vi "Database.Main.vi"() -> ()   [LabVIEW 2016]
uses:
  Database.Main.Action.ctl
  Database.Main.Data.ctl
  Database.Main.Data.Status.ctl
  Database.Main.Data.Sets.ctl
  Database.Main.Data.Results.ctl
  ProdaNG/Controls/ProdaNG.Identification.ctl
  ProdaNG/Controls/ProdaNG.ProcessResult.ctl
  ProdaNG/Controls/ProdaNG.ProcessStepResult.ctl
  ProdaNG/Controls/ProdaNG.TestStepResult.ctl
  ProdaNG/Controls/ProdaNG.TestValueResult.ctl
  Database.Main.Data.Variant.ctl
  ProdaNG/Controls/ProdaNG.ProcessStepParam.ctl
  ProdaNG/Controls/ProdaNG.TestStep.ctl
  ProdaNG/Controls/ProdaNG.TestStepParam.ctl
  ProdaNG/Controls/ProdaNG.TestValue.ctl
  tools/CitTemplate/citTemplate.errData.ctl
  tools/EventLog/EventLog.EventSource.ctl
  Databaser.SelectVariant.Format.ctl
  Logger/Logger.FileBody.ctl
  CheckStatusData.ctl
  Database.Global.vi
panel:
  out "Data out":T1 {"Variant"."TS"."TV"."minimum" format="%#.3f"; "Variant"."TS"."TV"."maximum" format="%#.3f"; "Variant"."TS"."TP"."value" format="%#.3f"}
  out "error.action":string
  out "error":errorcluster
  out "_loop":i32(ring)=4
  out "action":T15=enum."--- DB ---"
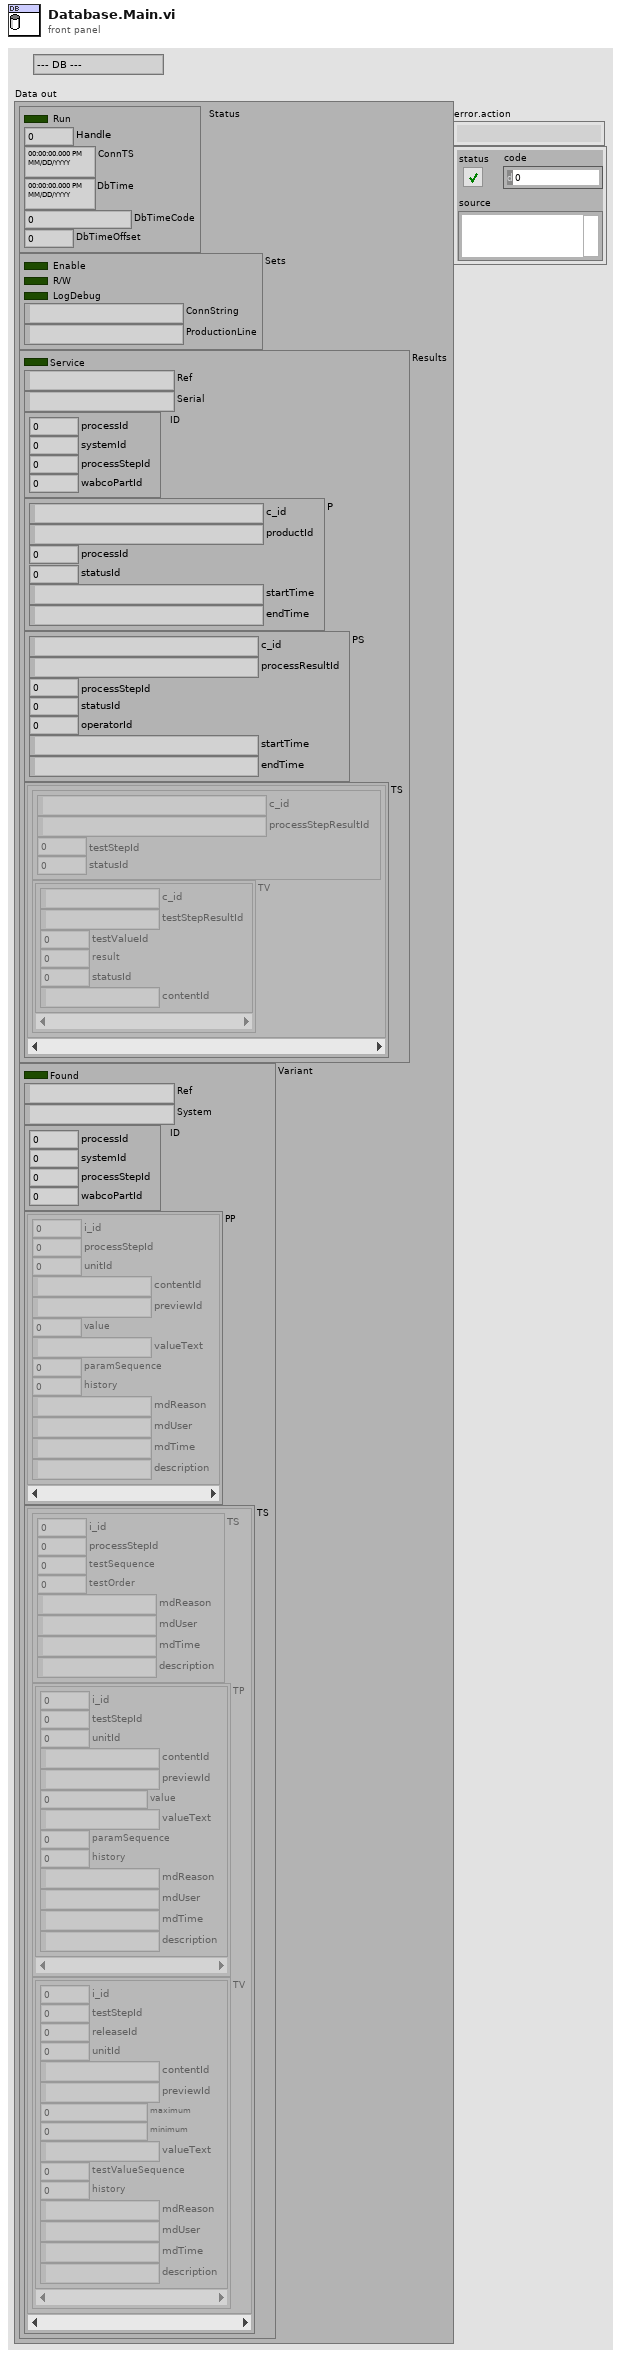
[diagram p1: front panel]
types:
  T1 = typedef "Database.Main.Data.ctl" = cluster{"Status":T2, "Sets":T3, "Results":T4, "Variant":T10}
  T2 = typedef "Database.Main.Data.Status.ctl" = cluster{"Run":bool, "Handle":i32, "ConnTS":timestamp, "DbTime":timestamp, "DbTimeCode":dbl, "DbTimeOffset":dbl}
  T3 = typedef "Database.Main.Data.Sets.ctl" = cluster{"Enable":bool, "R/W":bool, "LogDebug":bool, "ConnString":string, "ProductionLine":string}
  T4 = typedef "Database.Main.Data.Results.ctl" = cluster{"Service":bool, "Ref":string, "Serial":string, "ID":T5, "P":T6, "PS":T7, "TS":cluster{"TS":T8, "TV":T9[]}[]}
  T5 = typedef "ProdaNG.Identification.ctl" = cluster{"processId":i32, "systemId":i32, "processStepId":i32, "wabcoPartId":i32}
  T6 = typedef "ProdaNG.ProcessResult.ctl" = cluster{"c_id":string, "productId":string, "processId":i32, "statusId":i32, "startTime":string, "endTime":string}
  T7 = typedef "ProdaNG.ProcessStepResult.ctl" = cluster{"c_id":string, "processResultId":string, "processStepId":i32, "statusId":i32, "operatorId":i32, "startTime":string, "endTime":string}
  T8 = typedef "ProdaNG.TestStepResult.ctl" = cluster{"c_id":string, "processStepResultId":string, "testStepId":i32, "statusId":i32}
  T9 = typedef "ProdaNG.TestValueResult.ctl" = cluster{"c_id":string, "testStepResultId":string, "testValueId":i32, "result":dbl, "statusId":i32, "contentId":string}
  T10 = typedef "Database.Main.Data.Variant.ctl" = cluster{"Found":bool, "Ref":string, "System":string, "ID":T5, "PP":T11[], "TS":cluster{"TS":T12, "TP":T13[], "TV":T14[]}[]}
  T11 = typedef "ProdaNG.ProcessStepParam.ctl" = cluster{"i_id":i32, "processStepId":i32, "unitId":i32, "contentId":string, "previewId":string, "value":dbl, "valueText":string, "paramSequence":i32, "history":i32, "mdReason":string, "mdUser":string, "mdTime":string, "description":string}
  T12 = typedef "ProdaNG.TestStep.ctl" = cluster{"i_id":i32, "processStepId":i32, "testSequence":i32, "testOrder":i32, "mdReason":string, "mdUser":string, "mdTime":string, "description":string}
  T13 = typedef "ProdaNG.TestStepParam.ctl" = cluster{"i_id":i32, "testStepId":i32, "unitId":i32, "contentId":string, "previewId":string, "value":dbl, "valueText":string, "paramSequence":i32, "history":i32, "mdReason":string, "mdUser":string, "mdTime":string, "description":string}
  T14 = typedef "ProdaNG.TestValue.ctl" = cluster{"i_id":i32, "testStepId":i32, "releaseId":i32, "unitId":i32, "contentId":string, "previewId":string, "maximum":dbl, "minimum":dbl, "valueText":string, "testValueSequence":i32, "history":i32, "mdReason":string, "mdUser":string, "mdTime":string, "description":string}
  T15 = typedef "Database.Main.Action.ctl" = enum32{"idle", "constructor", "destructor", "--- DB ---", "Init", "Setup", "Select.Variant", "File.Export", "UpdateVariantFiles", "CheckStatus"}
  T16 = typedef "citTemplate.errData.ctl" = cluster{"ts":timestamp, "src":T17, "instance":i32, "action":string, "error":errorcluster, "unconfirmed":bool}
  T17 = typedef "EventLog.EventSource.ctl" = enum16{"All", "Gui", "Ref", "File", "Arch", "Seq", "CPX", "DB", "Laser", "Scan.P", "Scan.O", "PLC"}
  T18 = typedef "Databaser.SelectVariant.Format.ctl" = cluster{"System":string, "Variant":string}
  T19 = typedef "Logger.FileBody.ctl" = cluster{"Path":path, "System":string, "Status":u8, "Ref1":string, "Serial1":string, "Ref2":string, "Serial2":string, "Values":sgl[]}
  T20 = typedef "CheckStatusData.ctl" = cluster{"system":string, "Variant":string, "Serial":string}
  T21 = typedef "citTemplate.notifierHandle.ctl" = refnum<notifier>
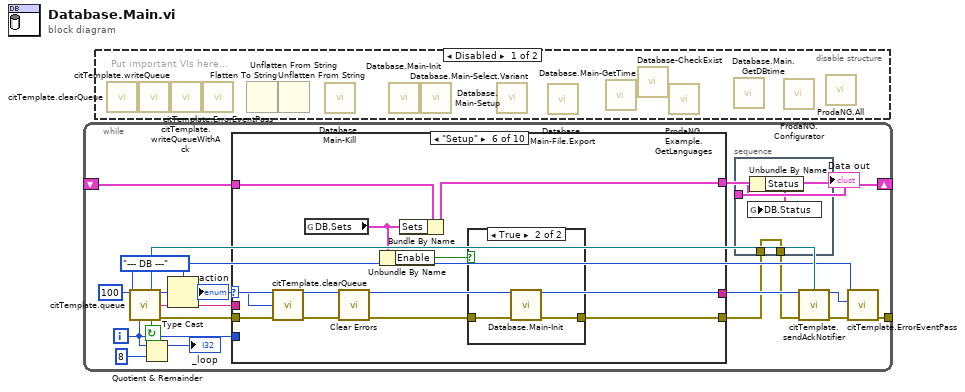
[diagram p0: block diagram]
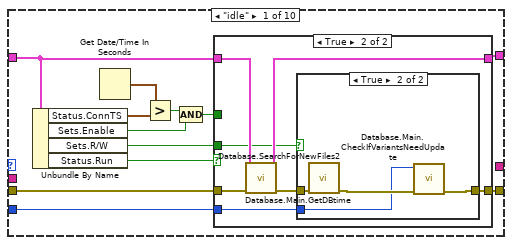
[diagram p3: hidden frame]
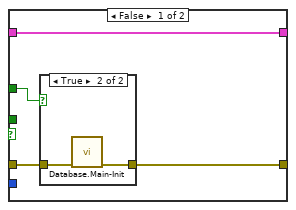
[diagram p4: hidden frame]
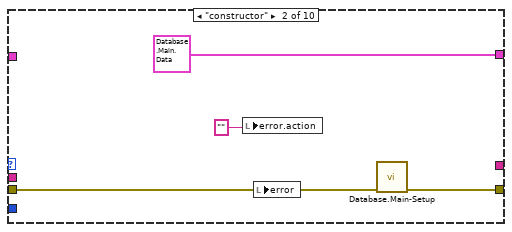
[diagram p7: hidden frame]
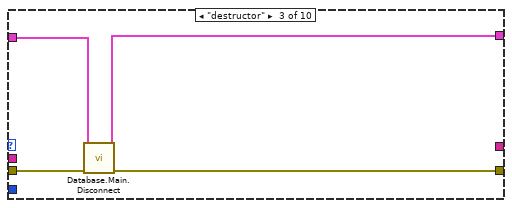
[diagram p8: hidden frame]
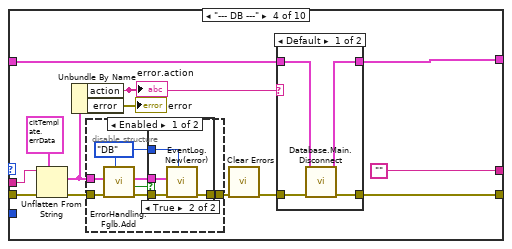
[diagram p9: hidden frame]
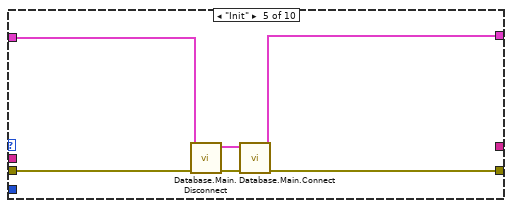
[diagram p13: hidden frame]
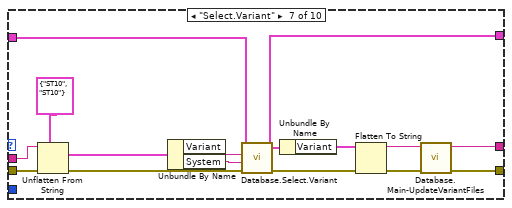
[diagram p15: hidden frame]
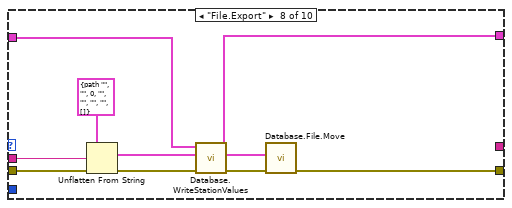
[diagram p16: hidden frame]
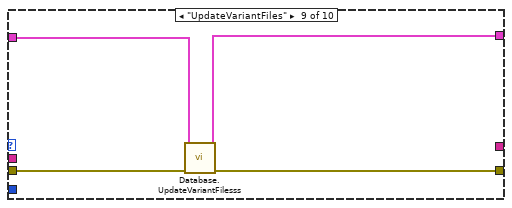
[diagram p17: hidden frame]
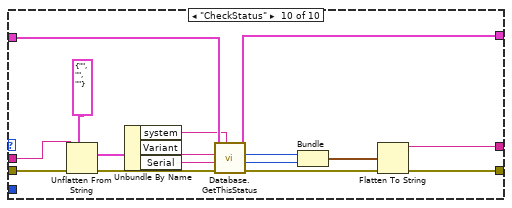
[diagram p18: hidden frame]
diagram:
  n1 = while {
    tunnel: [w12] -> _
    shift-right: [w2] -> _
    shift-left: _ -> [w3]
    i -> [w1]
    stop <- w14 continue-if-true
    w6 = Database.Main.Action."--- DB ---" ("Action")
    n2 = call "citTemplate.queue.vi"("ms timeout (250 ms)"=100, "event enum"=w6, "iteration (-1)"=w1) -> ("notifierHandle out"=w7:T21, "event out"=w17:u32, "(flatten) data out"=w16:string, "continue"=w14:bool, "error out"=w15:errorcluster)  [unwired: 2 in, 6 out]
    n3 = Quotient & Remainder(x=w1, y=8) -> (x-y*floor(x/y)=→"_loop":i32)  [unwired: 1 out]
    n4 = Type Cast(type=w6, x=w17) -> (*(type *) &x=w11:T15)
    "action" <- w11
    n5 = case shown="\"Setup\"" w11 {
      selector: w11 -> [_ _ _ _ _ w104 _ _ _ _]
      tunnel: w16 -> [_ _ _ w67 _ _ w121 w128 _ w136]
      tunnel: w15 -> [w30 w53 w59 w72 w94 w105 w122 w127 w135 w142]
      tunnel: [w27 w55 w58 w69 w96 w101 w113 w130 w134 w146] -> w5
      tunnel: w3 -> [w26 _ w57 w70 w93 w100 w119 w131 w133 w151]
      tunnel: [_ _ _ "" _ _ w117 _ _ w144] -> w8
      tunnel: [w22 T1 {"Status"={"Run"=FALSE, "Handle"=0, "ConnTS"=timestamp(0 s since 1904-01-01), "DbTime"=timestamp(0 s since 1904-01-01), "DbTimeCode"=0.0, "DbTimeOffset"=0.0}, "Sets"={"Enable"=FALSE, "R/W"=FALSE, "LogDebug"=FALSE, "ConnString"="", "ProductionLine"=""}, "Results"={"Service"=FALSE, "Ref"="", "Serial"="", "ID"={"processId"=0, "systemId"=0, "processStepId"=0, "wabcoPartId"=0}, "P"={"c_id"="", "productId"="", "processId"=0, "statusId"=0, "startTime"="", "endTime"=""}, "PS"={"c_id"="", "processResultId"="", "processStepId"=0, "statusId"=0, "operatorId"=0, "startTime"="", "endTime"=""}, "TS"=[]}, "Variant"={"Found"=FALSE, "Ref"="", "System"="", "ID"={"processId"=0, "systemId"=0, "processStepId"=0, "wabcoPartId"=0}, "PP"=[], "TS"=[]}} ("Data") w56 w60 w91 w97 w115 w123 w132 w150] -> w2
      tunnel: w1 -> [w21 _ _ _ _ _ _ _ _ _]
      frame "idle" {
        n6 = Unbundle By Name(w26) -> ("Status.ConnTS"=w31:timestamp, "Sets.Enable"=w24:bool, "Sets.R/W"=w23:bool, "Status.Run"=w28:bool)
        n7 = Get Date/Time In Seconds() -> (seconds since 1Jan1904=w32:timestamp)
        n8 = Greater?(x=w32, y=w31) -> (0:w29:bool)
        n9 = Compound Arithmetic op=AND(w29, w24) -> (w25:bool)
        n10 = case shown="True" w28 {
          tunnel: w30 -> [w36 w44]
          tunnel: w25 -> [w35 _]
          tunnel: [w34 w42] -> w27
          tunnel: w26 -> [w33 w46]
          tunnel: [w33 w45] -> w22
          tunnel: w23 -> [_ w41]
          tunnel: w21 -> [_ w40]
          frame False {
            n11 = case shown="True" w35 {
              tunnel: w36 -> [w37 w39]
              tunnel: [w37 w38] -> w34
              frame False {
              }
              frame True {
                n12 = call "Database.Main-Init.vi"("error in"=w39) -> ("error out"=w38:errorcluster)  [unwired: 10 in]
              }
            }
          }
          frame True {
            n13 = call "Database.Main.GetDBtime.vi"("error in (no error)"=w44, "Data in"=w46) -> ("error out"=w43:errorcluster, "Data out"=w45:T1)  [unwired: 8 in]
            n14 = case shown="True" w41 {
              tunnel: w43 -> [w47 w51]
              tunnel: [w47 w49] -> w42
              tunnel: w40 -> [_ w48]
              frame False {
              }
              frame True {
                n15 = call "Database.SearchForNewFiles2.vi"("error in"=w51) -> ("error out"=w50:errorcluster)  [unwired: 10 in]
                n16 = call "Database.Main.CheckIfVariantsNeedUpdate.vi"("error in (no error)"=w50, "i"=w48) -> ("error out"=w49:errorcluster)  [unwired: 9 in]
              }
            }
          }
        }
      }
      frame "constructor" {
        n17 = local write "error.action"("" ("error.action")) -> ()
        n18 = local write "error"(w53) -> ()
        n19 = call "Database.Main-Setup.vi"("error in"=w53) -> ("error out"=w55:errorcluster)  [unwired: 10 in]
      }
      frame "destructor" {
        n20 = call "Database.Main.Disconnect.vi"("error in (no error)"=w59, "Data"=w57) -> ("error out"=w58:errorcluster, "DataOut"=w56:T1)  [unwired: 8 in]
      }
      frame "--- DB ---" {
        n21 = Unflatten From String(type=T16 {"ts"=timestamp(0 s since 1904-01-01), "src"=enum."All", "instance"=0, "action"="", "error"={"status"=FALSE, "code"=0, "source"=""}, "unconfirmed"=FALSE} ("ErrData"), binary string=w67, error in (no error)=w72) -> (value=w62:T16, error out=w65:errorcluster)  [unwired: 3 out]
        n22 = Unbundle By Name(w62) -> ("action"=w61:string, "error"=→"error":errorcluster)
        "error.action" <- w61
        n23 = disable-structure shown="Enabled" {
          disable-tunnel: w65 -> [w76 w84]
          disable-tunnel: [w74 w84] -> w64
          disable-tunnel: w62 -> [w73 _]
          frame Enabled {
            w75 = EventLog.EventSource."DB" ("Event source")
            n24 = call "ErrorHandling.Fglb.Add.vi"("Event source"=w75, "error in (no error)"=w76, "Error in"=w73) -> ("error out"=w78:errorcluster, "changed?"=w77:bool)  [unwired: 7 in]
            n25 = case shown="True" w77 {
              tunnel: [w79 w83] -> w74
              tunnel: w73 -> [_ w82]
              tunnel: w78 -> [w79 w81]
              tunnel: w75 -> [_ w80]
              frame False {
              }
              frame True {
                n26 = call "EventLog.New(error).vi"("Source (All)"=w80, "error in"=w81, "ErrData"=w82) -> ("error out"=w83:errorcluster)  [unwired: 8 in]
              }
            }
          }
          frame Disabled {
          }
        }
        n27 = call <vilib>:"Clear Errors.vi"("error in (no error)"=w64) -> ("error out"=w68:errorcluster)  [unwired: 5 in, 1 out]
        n28 = case shown="Default" w61 {
          tunnel: w70 -> [w88 w89]
          tunnel: [w87 w89] -> w60
          tunnel: [w86 w90] -> w69
          tunnel: w68 -> [w85 w90]
          frame Default {
            n29 = call "Database.Main.Disconnect.vi"("error in (no error)"=w85, "Data"=w88) -> ("error out"=w86:errorcluster, "DataOut"=w87:T1)  [unwired: 8 in]
          }
          frame "Process File" {
          }
        }
      }
      frame "Init" {
        n30 = call "Database.Main.Disconnect.vi"("error in (no error)"=w94, "Data"=w93) -> ("error out"=w95:errorcluster, "DataOut"=w92:T1)  [unwired: 8 in]
        n31 = call "Database.Main.Connect.vi"("error in (no error)"=w95, "Data in"=w92) -> ("error out"=w96:errorcluster, "Data out"=w91:T1)  [unwired: 8 in]
      }
      frame "Setup" {
        n32 = call "citTemplate.clearQueue.vi"("event in"=w104, "error in (no error)"=w105) -> ("error out"=w103:errorcluster)  [unwired: 12 in, 1 out]
        n33 = global read "Database.Global.vi" "DB.Sets"() -> (w99:T3)
        n34 = call <vilib>:"Clear Errors.vi"("error in (no error)"=w103) -> ("error out"=w102:errorcluster)  [unwired: 5 in, 1 out]
        n35 = Unbundle By Name(w99) -> ("Enable"=w98:bool)
        n36 = Bundle By Name(cluster=w100, "Sets"=w99) -> (w97:T1)
        n37 = case shown="True" w98 {
          tunnel: w102 -> [w106 w108]
          tunnel: [w106 w107] -> w101
          frame False {
          }
          frame True {
            n38 = call "Database.Main-Init.vi"("error in"=w108) -> ("error out"=w107:errorcluster)  [unwired: 10 in]
          }
        }
      }
      frame "Select.Variant" {
        n39 = Unflatten From String(type=T18 {"System"="ST10", "Variant"="ST10"}, binary string=w121, error in (no error)=w122) -> (value=w111:T18, error out=w120:errorcluster)  [unwired: 3 out]
        n40 = Unbundle By Name(w111) -> ("Variant"=w110:string, "System"=w109:string)
        n41 = call "Database.Select.Variant.vi"("error in"=w120, "System"=w109, "Variant"=w110, "Data in"=w119) -> ("error out"=w118:errorcluster, "Data out"=w115:T1)  [unwired: 6 in]
        n42 = Unbundle By Name(w115) -> ("Variant"=w116:T10)
        n43 = Flatten To String(anything=w116, error in (no error)=w118) -> (data string=w117:string, error out=w114:errorcluster)  [unwired: 2 in, 1 out]
        n44 = call "Database.Main-UpdateVariantFiles.vi"("error in"=w114) -> ("error out"=w113:errorcluster)  [unwired: 10 in]
      }
      frame "File.Export" {
        n45 = Unflatten From String(type=T19 {"Path"=path "", "System"="", "Status"=0, "Ref1"="", "Serial1"="", "Ref2"="", "Serial2"="", "Values"=[]} ("FileBody"), binary string=w128, error in (no error)=w127) -> (value=w124:T19, error out=w125:errorcluster)  [unwired: 2 in, 1 out]
        n46 = call "Database.WriteStationValues.vi"("error in"=w125, "FileBody"=w124, "Data in"=w131) -> ("error out"=w129:errorcluster, "Data out"=w123:T1)  [unwired: 7 in]
        n47 = call "Database.File.Move.vi"("error in (no error)"=w129, "FileBody"=w124) -> ("error out"=w130:errorcluster)  [unwired: 9 in]
      }
      frame "UpdateVariantFiles" {
        n48 = call "Database.UpdateVariantFilesss.vi"("error in (no error)"=w135, "Data in"=w133) -> ("error out"=w134:errorcluster, "Data out"=w132:T1)  [unwired: 8 in]
      }
      frame "CheckStatus" {
        n49 = Unflatten From String(type=T20 {"system"="", "Variant"="", "Serial"=""} ("CheckStatusData"), binary string=w136, error in (no error)=w142) -> (value=w141:T20, error out=w137:errorcluster)  [unwired: 2 in, 1 out]
        n50 = Unbundle By Name(w141) -> ("system"=w140:string, "Variant"=w139:string, "Serial"=w138:string)
        n51 = call "Database.GetThisStatus.vi"("system"=w140, "error in"=w137, "Serial"=w138, "Variant"=w139, "Data in"=w151) -> ("error out"=w147:errorcluster, "Repetitions"=w148:u8, "Status"=w149:i8, "Data out"=w150:T1)  [unwired: 3 in]
        n52 = Bundle("Status"=w149, "Repetitions"=w148) -> (w145:cluster{"Status":i8, "Repetitions":u8})  [unwired: 1 in]
        n53 = Flatten To String(anything=w145, error in (no error)=w147) -> (data string=w144:string, error out=w146:errorcluster)  [unwired: 2 in, 1 out]
      }
    }
    "Data out" <- w2
    n54 = stacked-sequence {
      tunnel: w2 -> [w20]
      tunnel: [w18] -> w4
      tunnel: w5 -> [w18]
      frame #0 {
        n55 = Unbundle By Name(w20) -> ("Status"=w19:T2)
        n56 = global write "Database.Global.vi" "DB.Status"(w19) -> ()
      }
    }
    n57 = call "citTemplate.sendAckNotifier.vi"("notification data"=w8, "notifierHandle in"=w7, "error in"=w4) -> ()  [unwired: 13 in]
    n58 = call "citTemplate.ErrorEventPass.vi"("error in"=w4, "action of error"=w11, "event in"=w6) -> ("error out"=w12:errorcluster)  [unwired: 2 in, 6 out]
  }
  n59 = disable-structure shown="Disabled" {
    frame Disabled {
      # "Put important VIs here..."
      n60 = call "citTemplate.clearQueue.vi"() -> ()  [unwired: 14 in, 2 out]
      n61 = call "citTemplate.writeQueue.vi"() -> ()  [unwired: 15 in, 1 out]
      n62 = call "citTemplate.writeQueueWithAck.vi"() -> ()  [unwired: 13 in, 3 out]
      n63 = call "citTemplate.ErrorEventPass.vi"() -> ()  [unwired: 11 in, 1 out]
      n64 = Flatten To String() -> ()  [unwired: 4 in, 3 out]
      n65 = Unflatten From String() -> ()  [unwired: 5 in, 3 out]
      n66 = Unflatten From String() -> ()  [unwired: 5 in, 3 out]
      n67 = call "Database.Main-Kill.vi"() -> ()  [unwired: 11 in, 1 out]
      n68 = call "Database.Main-Init.vi"() -> ()  [unwired: 11 in, 1 out]
      n69 = call "Database.Main-Setup.vi"() -> ()  [unwired: 11 in, 1 out]
      n70 = call "Database.Main-Select.Variant.vi"() -> ()  [unwired: 11 in, 1 out]
      n71 = call "Database.Main-File.Export.vi"() -> ()  [unwired: 11 in, 1 out]
      n72 = call "Database.Main-GetTime.vi"() -> ()  [unwired: 1 in, 1 out]
      n73 = call "Database-CheckExist.vi"() -> ()  [unwired: 9 in, 3 out]
      n74 = call "ProdaNG.Example.GetLanguages.vi"() -> ()  [unwired: 12 in]
      n75 = call "Database.Main.GetDBtime.vi"() -> ()  [unwired: 10 in, 2 out]
      n76 = call "ProdaNG.Configurator.vi"() -> ()  [unwired: 12 in]
      n77 = call "ProdaNG.All.vi"() -> ()  [unwired: 12 in]
    }
    frame Enabled {
    }
  }
